vi "loadHolo.vi"(4 "Display":u8, 7 "Cluster":T1, 8 "Image":T2) -> (1 "Y position":dbl, 2 "X position":dbl, 3 "CGH":T2(plugin-control))   [LabVIEW 2022 SP3]
uses:
  <vilib>/vision/Image Controls.llb/IMAQ Image.ctl
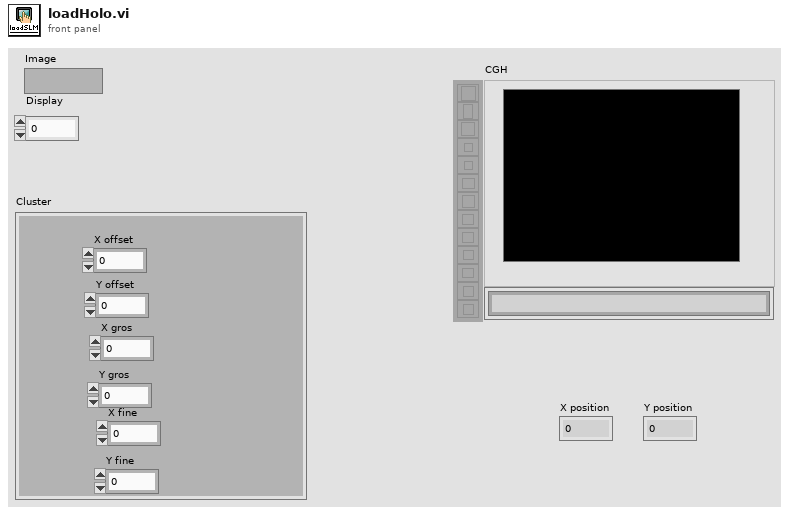
[diagram p1: front panel]
types:
  T1 = cluster{"X offset":dbl, "Y offset":dbl, "X gros":dbl, "Y gros":dbl, "X fine":dbl, "Y fine":dbl}
  T2 = typedef "IMAQ Image.ctl" = refnum<image>
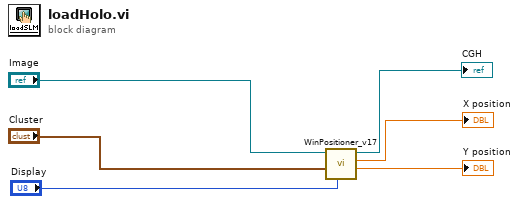
[diagram p0: block diagram]
diagram:
  n1 = call "WinPositioner_v17.vi"("Display (1, 2...)"="Display", "Cluster"="Cluster", "Image"="Image") -> ("Y position"=→"Y position":dbl, "X position"=→"X position":dbl, "CGH_x"=→"CGH":T2)  [unwired: 6 in]
